vi "Config Type.vi"(11 "Stop Seq Command in":refnum<class "Stop Seq Command.lvclass">) -> (2 "Command Config Type":refnum<class "Command Config.lvclass">)   [LabVIEW 2020, in "VolatusSeq.lvlib" / "Stop Seq Command.lvclass"]
uses:
  Stop Seq Command.lvclass
  VolatusSeqConfig/Command Config/Command Config.lvclass
  VolatusSeqConfig/Stop Seq Command Config/Stop Seq Command Config.lvclass
  C:/dev/lv20CE/relink/lv-volatus/VolatusSeqConfig/Command Config/Command Config.lvclass
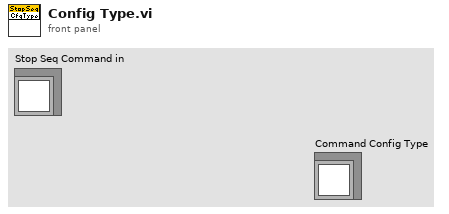
[diagram p1: front panel]
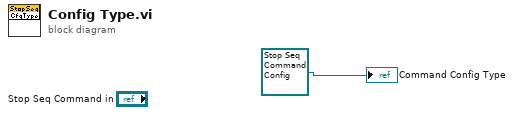
[diagram p0: block diagram]
diagram:
  "Command Config Type" <- refnum<class "Stop Seq Command Config.lvclass"> refnum ("VolatusSeqConfig.lvlib:Stop Seq Command Config.lvclass")
